vi "test1_160531.vi"() -> ()   [LabVIEW 2015]
uses:
  <vilib>/NXT/Block Support/NXT_OutputPort.ctl
  <vilib>/NXT/Block Support/NXT_InputPort.ctl
  <vilib>/NXT/NXTIO Xnodes/NXTIONodeSubVIs/NXTMoveMotors.vi
  <vilib>/NXT/Dual Mode Library/Waits/Wait_Num.vi
  <vilib>/NXT/Dual Mode Library/Sensors/Light_On.vi
  <vilib>/NXT/Dual Mode Library/Sensors/Touch_Pressed.vi
  <vilib>/NXT/Dual Mode Library/Sensors/Sonar_cm.vi
  <vilib>/NXT/Subs/LVHSConnector.ctl
  <vilib>/NXT/NXTIO Xnodes/AddressXNode/NXTIOAddress.xnode
  <vilib>/NXT/NXTIO Xnodes/NXTIOXNode/NXTIO.xnode
  <vilib>/NXT/LegoClasses/BrickReference/BrickReference.lvclass
panel:
  in  "startright/Speed 2":i8=75
  in  "startrightB/Speed 1":i8=75
  in  "turn lefttC 2":i8=75
  in  "turn lefttB 2":i8=75
  in  "Go-ahead":i8=75
  out "check destance":i16(slide) scale=0.0..100.0
  in  "turn rightC":i8=75
  in  "turn rightB":i8=75
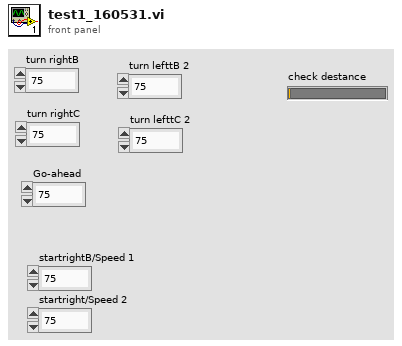
[diagram p1: front panel]
types:
  T1 = typedef "NXT_OutputPort.ctl" = u8
  T2 = typedef "LVHSConnector.ctl" = refnum<class "BrickReference.lvclass">
  T3 = typedef "NXT_InputPort.ctl" = u32
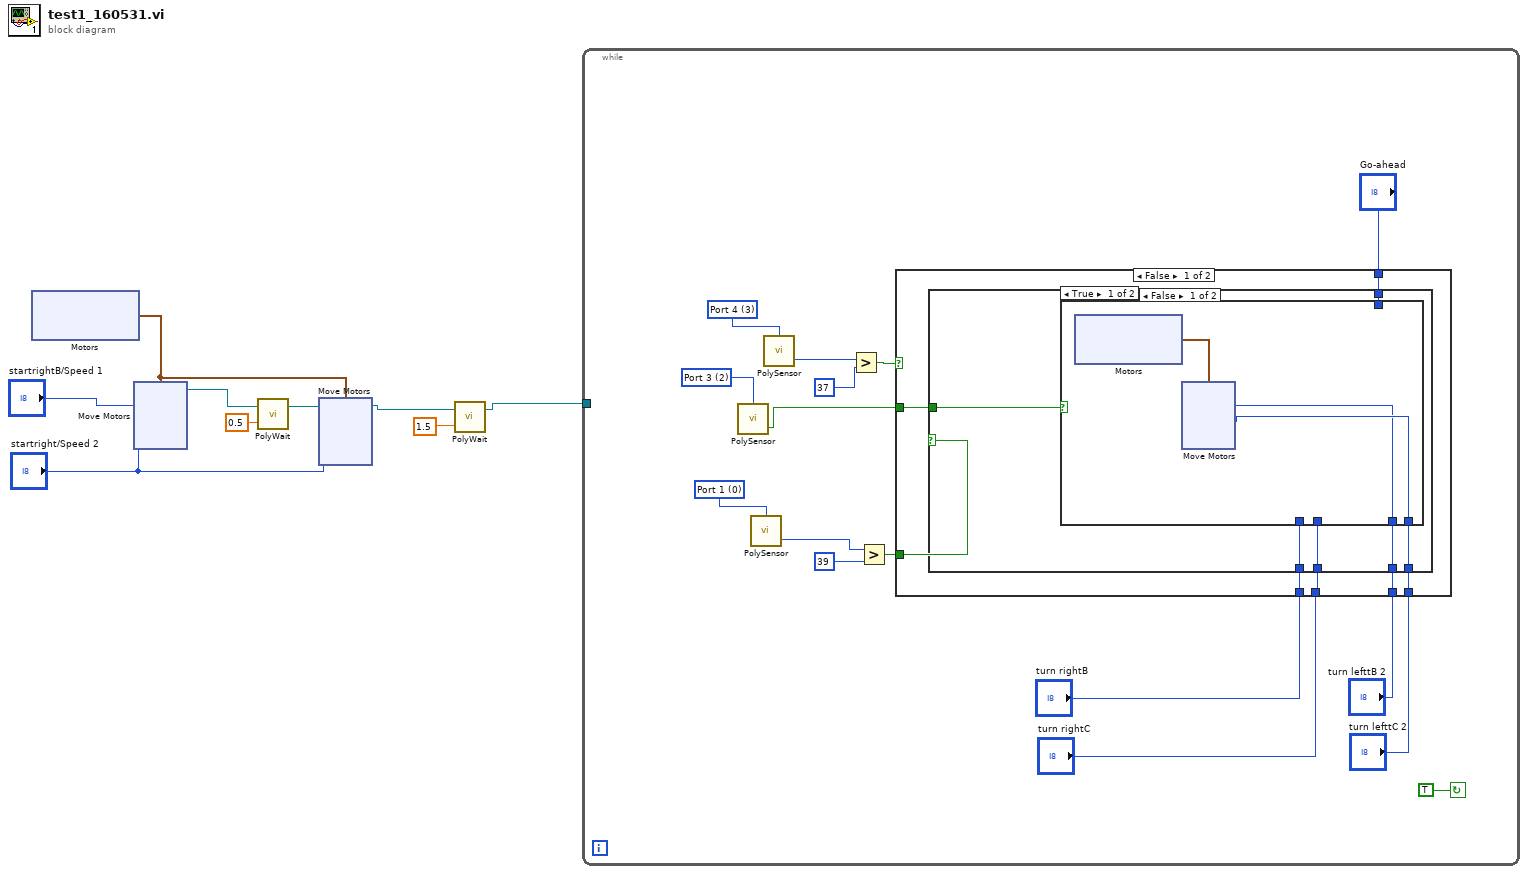
[diagram p0: block diagram]
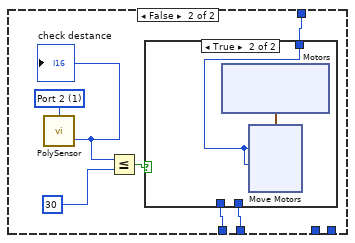
[diagram p2: hidden frame]
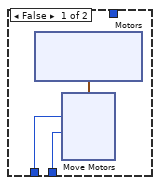
[diagram p3: hidden frame]
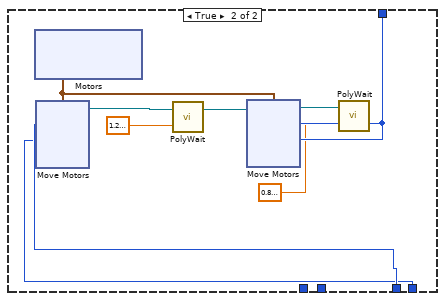
[diagram p4: hidden frame]
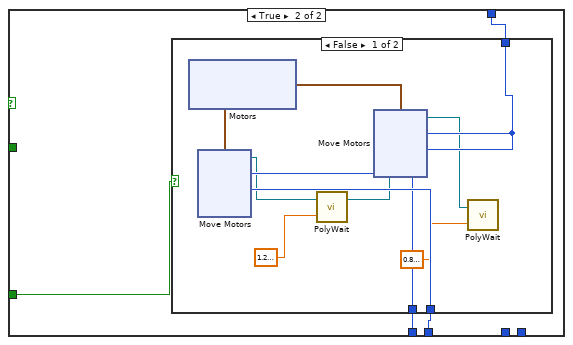
[diagram p5: hidden frame]
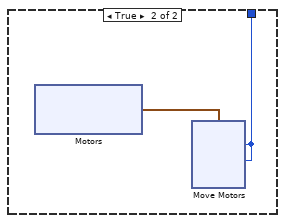
[diagram p6: hidden frame]
diagram:
  n1 = xnode "Motors"() -> ("Motor"=w7:cluster{"Port":T1, "Port":T1})
  n2 = xnode "Move Motors"("Power/Speed 2"="startright/Speed 2", "Power/Speed 1"="startrightB/Speed 1", "Motors"=w7) -> ("NXT/EV3"=w8:T2)  [unwired: 1 in]
  n3 = call-poly <vilib>:"PolyWait.vi"("Time (1 sec)"=sgl 0.5, "NXT/EV3"=w8) -> ("NXT/EV3"=w6:T2)  [unwired: 2 in]
  n4 = xnode "Move Motors"("Power/Speed 2"="startright/Speed 2", "Power/Speed 1"="startright/Speed 2", "Motors"=w7, "NXT/EV3"=w6) -> ("NXT/EV3"=w4:T2)
  n5 = call-poly <vilib>:"PolyWait.vi"("Time (1 sec)"=sgl 1.5, "NXT/EV3"=w4) -> ("NXT/EV3"=w3:T2)  [unwired: 2 in]
  n6 = while {
    tunnel: w3 -> [_]
    stop <- TRUE continue-if-true
    w10 = T3 2 items=["Port 1", "Port 2", "Port 3", "Port 4"] ("Port (Port 1)")
    w21 = T3 3 items=["Port 1", "Port 2", "Port 3", "Port 4"] ("Port (Port 3)")
    w20 = T3 0 items=["Port 1", "Port 2", "Port 3", "Port 4"] ("Port (Port 3)")
    n7 = call-poly <vilib>:"PolySensor.vi"("Port (Port 1)"=w10) -> ("Yes / No"=w11:bool)  [unwired: 2 in, 1 out]
    n8 = call-poly <vilib>:"PolySensor.vi"("Port (Port 3)"=w20) -> ("Scaled Value"=w22:i16)  [unwired: 2 in, 1 out]
    n9 = call-poly <vilib>:"PolySensor.vi"("Port (Port 3)"=w21) -> ("Scaled Value"=w24:i16)  [unwired: 2 in, 1 out]
    n10 = Greater?(x=w24, y=i16 37) -> (0:w19:bool)
    n11 = Greater?(x=w22, y=i16 39) -> (0:w18:bool)
    n12 = case shown="False" w19 {
      tunnel: w18 -> [w32 w110]
      tunnel: "turn rightB" -> [w31 w109]
      tunnel: "turn rightC" -> [w30 w108]
      tunnel: "Go-ahead" -> [w29 w107]
      tunnel: "turn lefttB 2" -> [w28 _]
      tunnel: "turn lefttC 2" -> [w27 _]
      tunnel: w11 -> [w26 _]
      frame False {
        n13 = case shown="False" w32 {
          tunnel: w31 -> [w38 _]
          tunnel: w30 -> [w37 _]
          tunnel: w29 -> [w36 w85]
          tunnel: w28 -> [w34 w89]
          tunnel: w27 -> [w33 w88]
          tunnel: w26 -> [w35 _]
          frame False {
            n14 = case shown="True" w35 {
              tunnel: w38 -> [_ w57]
              tunnel: w37 -> [_ w56]
              tunnel: w36 -> [_ w51]
              tunnel: w34 -> [w39 _]
              tunnel: w33 -> [w40 _]
              frame True {
                n15 = xnode "Motors"() -> ("Motor"=w41:cluster{"Port":T1, "Port":T1})
                n16 = xnode "Move Motors"("Power/Speed 2"=w40, "Power/Speed 1"=w39, "Motors"=w41) -> ()  [unwired: 1 in, 1 out]
              }
              frame False {
                w54 = T3 1 items=["Port 1", "Port 2", "Port 3", "Port 4"] ("Port (Port 4)")
                n17 = call-poly <vilib>:"PolySensor.vi"("Port (Port 4)"=w54) -> ("Distance (cm)"=w55:i16)  [unwired: 2 in, 1 out]
                "check destance" <- w55
                n18 = Less Or Equal?(x=w55, y=i16 30) -> (x <= y?=w52:bool)
                n19 = case shown="True" w52 {
                  tunnel: w57 -> [w59 _]
                  tunnel: w56 -> [w58 _]
                  tunnel: w51 -> [_ w70]
                  frame False {
                    n20 = xnode "Motors"() -> ("Motor"=w60:cluster{"Port":T1, "Port":T1})
                    n21 = xnode "Move Motors"("Power/Speed 2"=w58, "Power/Speed 1"=w59, "Motors"=w60) -> ()  [unwired: 1 in, 1 out]
                  }
                  frame True {
                    n22 = xnode "Motors"() -> ("Motor"=w71:cluster{"Port":T1, "Port":T1})
                    n23 = xnode "Move Motors"("Power/Speed 2"=w70, "Power/Speed 1"=w70, "Motors"=w71) -> ()  [unwired: 1 in, 1 out]
                  }
                }
              }
            }
          }
          frame True {
            n24 = xnode "Motors"() -> ("Motor"=w86:cluster{"Port":T1, "Port":T1})
            n25 = xnode "Move Motors"("Power/Speed 2"=w88, "Power/Speed 1"=w89, "Motors"=w86) -> ("NXT/EV3"=w87:T2)  [unwired: 1 in]
            n26 = call-poly <vilib>:"PolyWait.vi"("Time (1 sec)"=sgl 1.3, "NXT/EV3"=w87) -> ("NXT/EV3"=w84:T2)  [unwired: 2 in]
            n27 = xnode "Move Motors"("Power/Speed 2"=w85, "Power/Speed 1"=w85, "Motors"=w86, "NXT/EV3"=w84) -> ("NXT/EV3"=w83:T2)
            n28 = call-poly <vilib>:"PolyWait.vi"("Time (1 sec)"=sgl 0.8, "NXT/EV3"=w83) -> ()  [unwired: 2 in, 1 out]
          }
        }
      }
      frame True {
        n29 = case shown="False" w110 {
          tunnel: w109 -> [w118 _]
          tunnel: w108 -> [w119 _]
          tunnel: w107 -> [w116 w137]
          frame False {
            n30 = xnode "Motors"() -> ("Motor"=w117:cluster{"Port":T1, "Port":T1})
            n31 = xnode "Move Motors"("Power/Speed 2"=w119, "Power/Speed 1"=w118, "Motors"=w117) -> ("NXT/EV3"=w115:T2)  [unwired: 1 in]
            n32 = call-poly <vilib>:"PolyWait.vi"("Time (1 sec)"=sgl 1.3, "NXT/EV3"=w115) -> ("NXT/EV3"=w114:T2)  [unwired: 2 in]
            n33 = xnode "Move Motors"("Power/Speed 2"=w116, "Power/Speed 1"=w116, "Motors"=w117, "NXT/EV3"=w114) -> ("NXT/EV3"=w113:T2)
            n34 = call-poly <vilib>:"PolyWait.vi"("Time (1 sec)"=sgl 0.8, "NXT/EV3"=w113) -> ()  [unwired: 2 in, 1 out]
          }
          frame True {
            n35 = xnode "Motors"() -> ("Motor"=w138:cluster{"Port":T1, "Port":T1})
            n36 = xnode "Move Motors"("Power/Speed 2"=w137, "Power/Speed 1"=w137, "Motors"=w138) -> ()  [unwired: 1 in, 1 out]
          }
        }
      }
    }
  }
